vi "BORRADO_MEJORADO.vi"(9 "MB LIBRE OK":i64, 11 "MB Minimo de Memoria libre":i64) -> ()   [LabVIEW 2015]
panel:
  out "deleted path":path
  out "x > y?":bool
  out "deleted portion":path
  out "last mod":timestamp
  in  "error in":errorcluster
  out "error out 2":errorcluster
  out "Array 4":bool[](array[boolean])
  out "All Files in Dir 4":path[](array[path])
  out "double precision float 6":dbl
  out "double precision float 5":dbl
  out "x-y 3":dbl
  out "date string 3":string
  out "time string 5":string
  out "time string 7":string
  out "Array 3":timestamp[](array[timestamp])
  out "size 3":i64
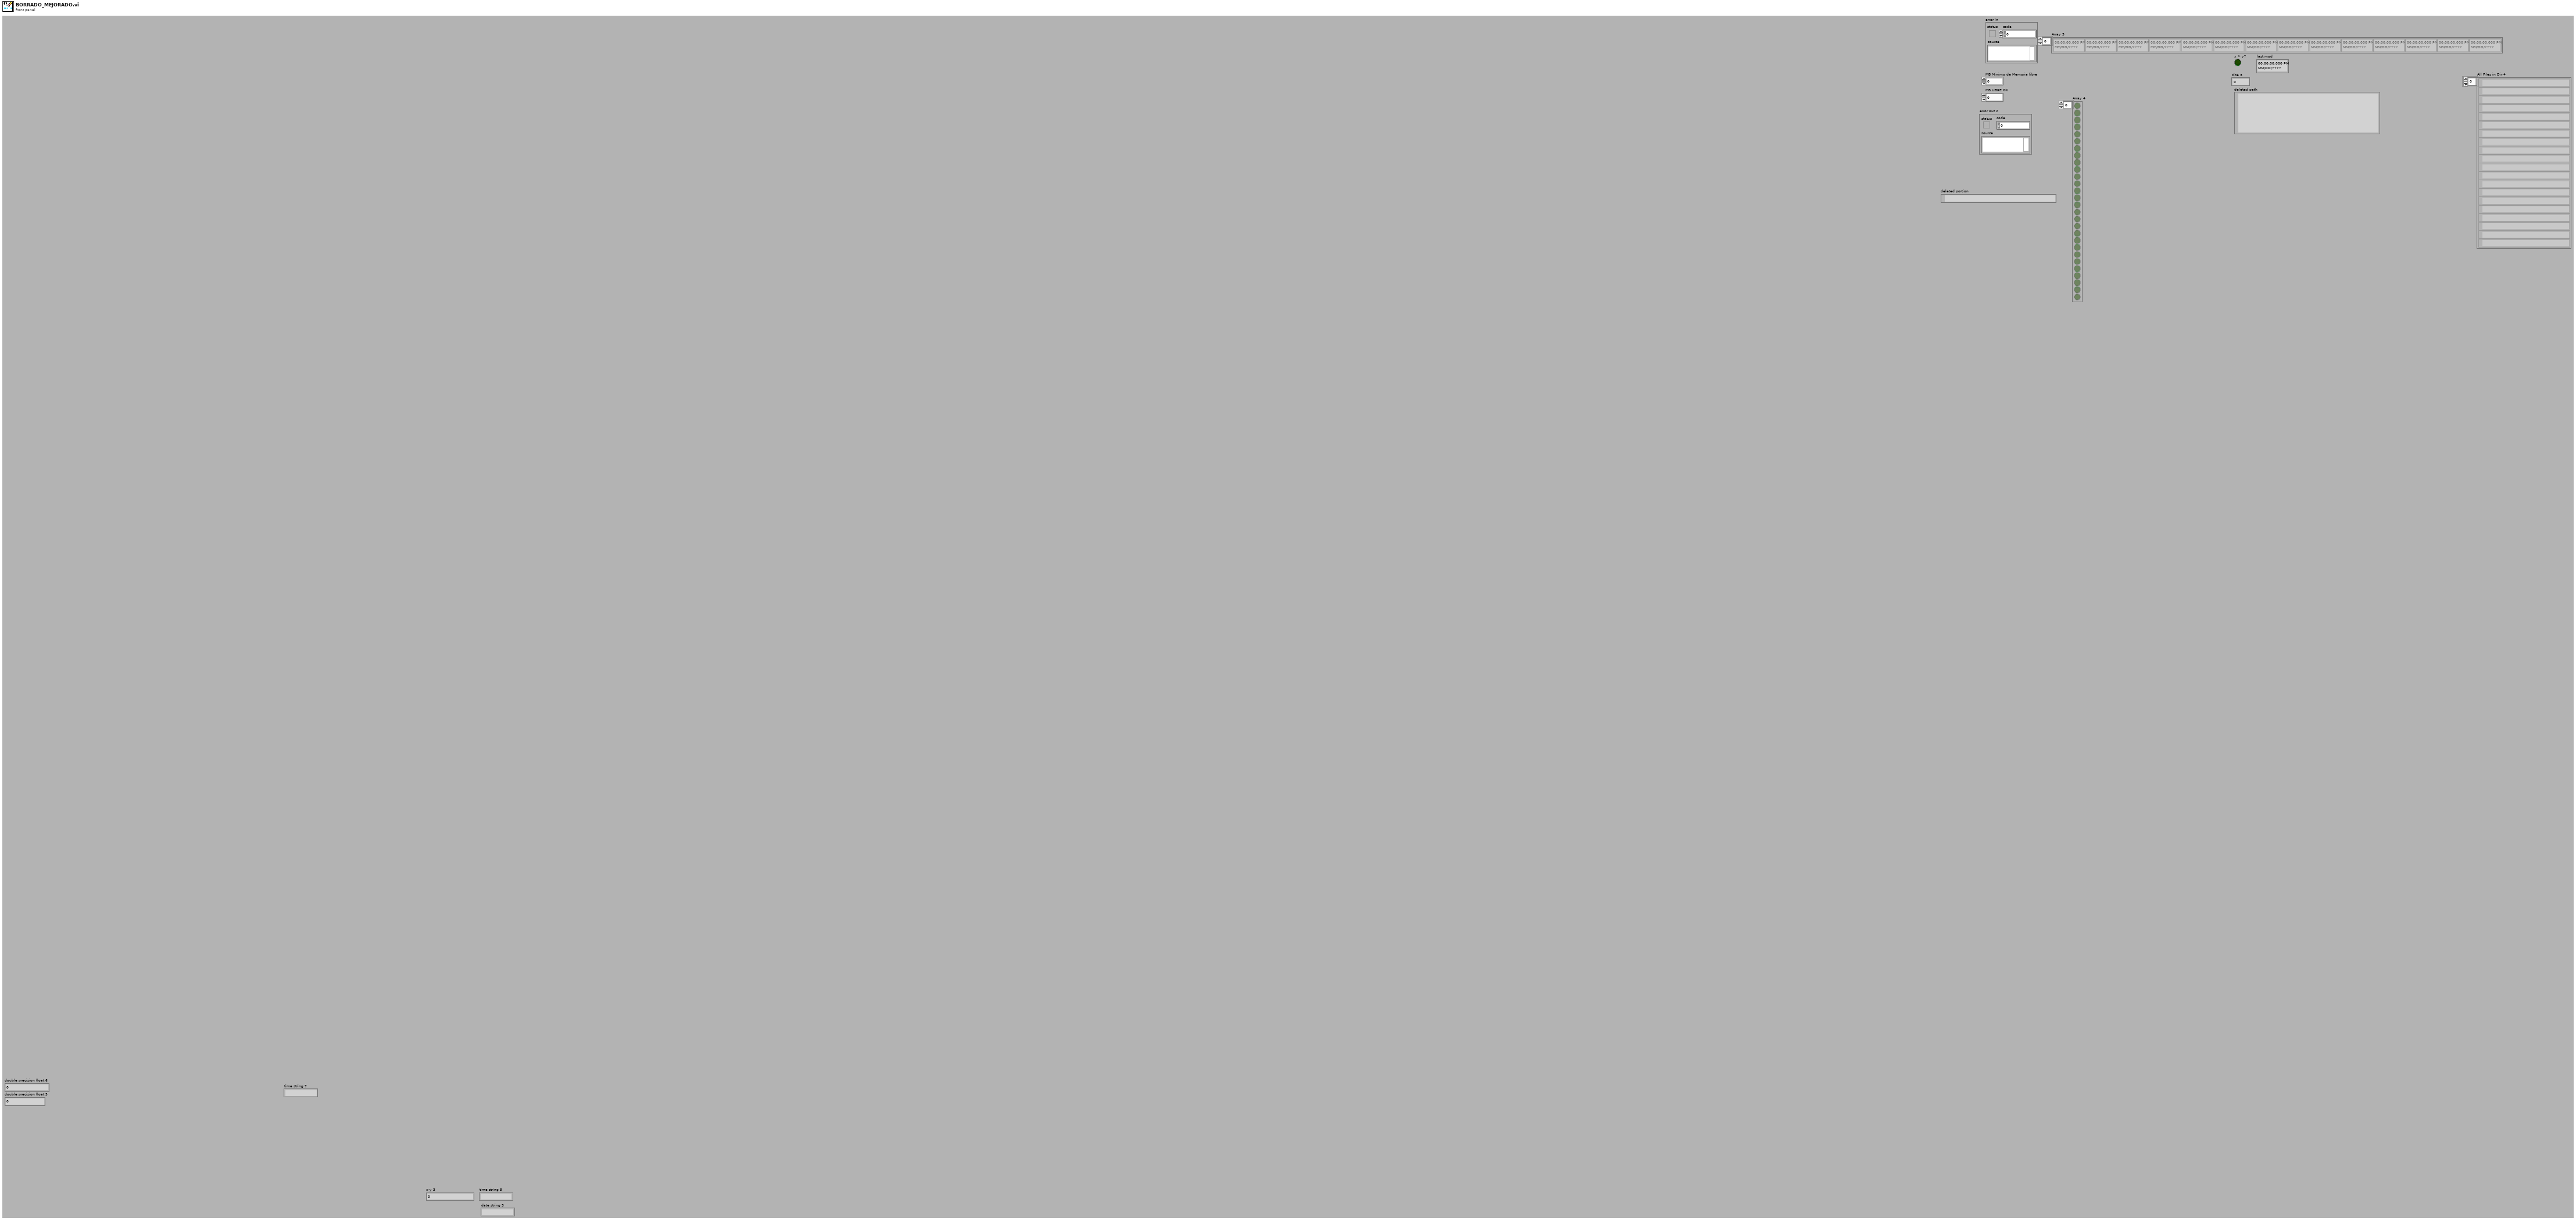
[diagram p1: front panel]
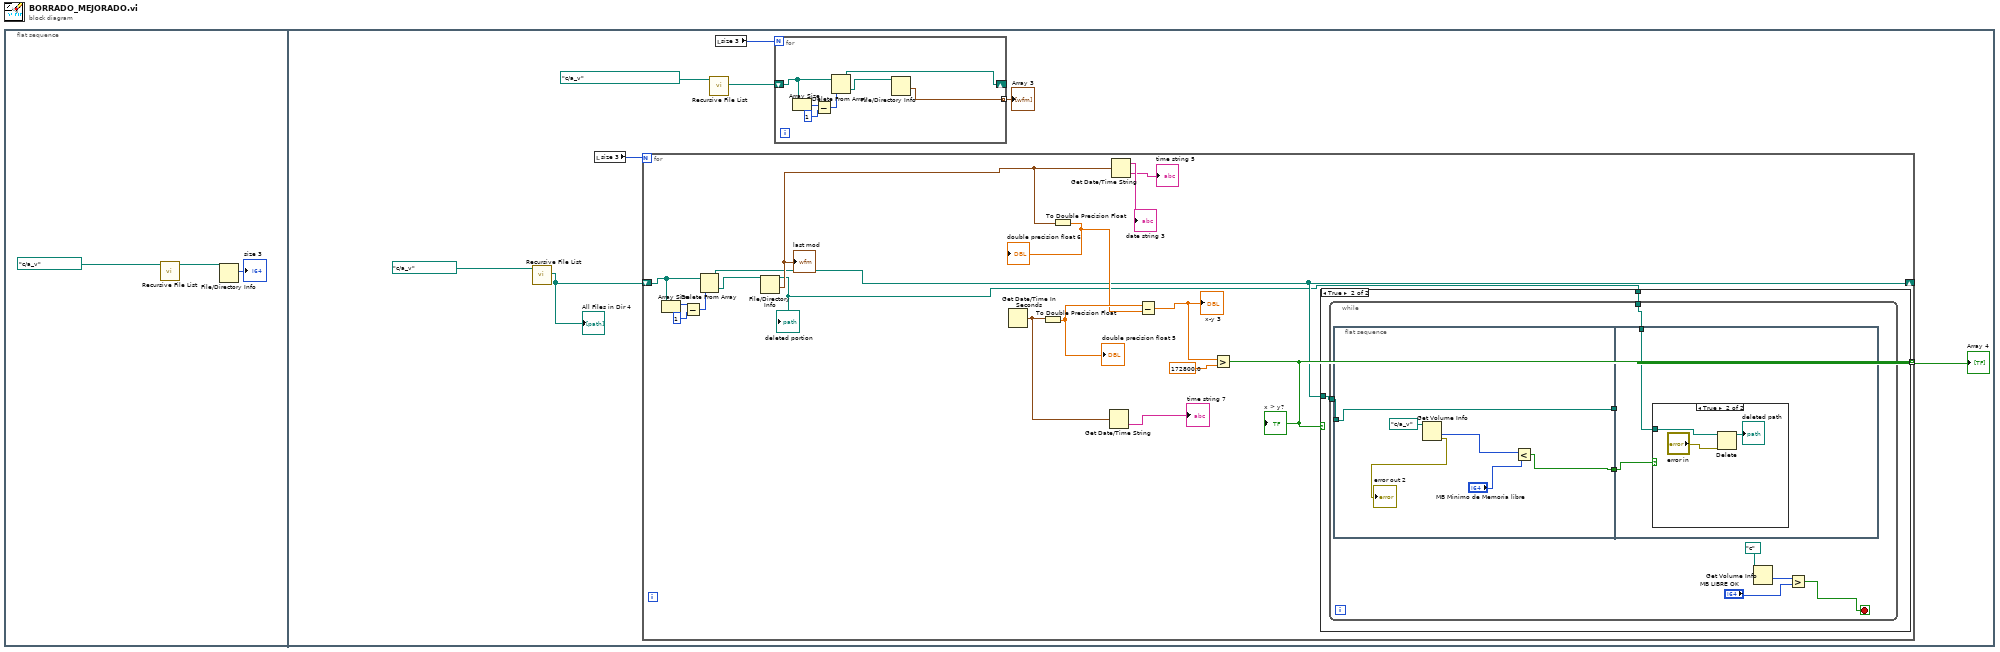
[diagram p0: block diagram]
diagram:
  n1 = flat-sequence {
    frame #0 {
      n2 = call <vilib>:"Recursive File List.vi"("Folder Path"=path "c:/a_v" ("path")) -> ("dup Folder Path"=w2:path)  [unwired: 6 in, 4 out]
      n3 = File/Directory Info(path=w2) -> (size=→"size 3":i64)  [unwired: 1 in, 6 out]
    }
    frame #1 {
      n4 = call <vilib>:"Recursive File List.vi"("Folder Path"=path "c:/a_v" ("path")) -> ("All Files in Dir"=w9:path[])  [unwired: 6 in, 4 out]
      "All Files in Dir 4" <- w9
      n5 = local read "size 3"() -> (w11:i64)
      n6 = for {
        N: w11 -> [_]
        shift-right: [w13] -> _
        shift-left: w9 -> [w24]
        tunnel: [w14] -> w10 mode=indexing
        n7 = Array Size(array=w24) -> (size(s)=w25:i32)
        n8 = Subtract(x=w25, y=1 ("length")) -> (x-y=w27:i32)
        n9 = Delete From Array(array=w24, index=w27) -> (deleted portion=w12:path, array with subset deleted=w13:path[])  [unwired: 1 in]
        "deleted portion" <- w12
        n10 = File/Directory Info(path=w12) -> (last mod=w15:timestamp)  [unwired: 1 in, 6 out]
        "last mod" <- w15
        n11 = Get Date/Time In Seconds() -> (seconds since 1Jan1904=w19:timestamp)
        n12 = To Double Precision Float(number=w19) -> (double precision float=w22:dbl)
        "double precision float 5" <- w22
        n13 = To Double Precision Float(number=w15) -> (double precision float=w21:dbl)
        "double precision float 6" <- w21
        n14 = Get Date/Time String(seconds (now)=w19) -> (time string=→"time string 7":string)  [unwired: 2 in, 1 out]
        n15 = Get Date/Time String(seconds (now)=w15) -> (date string=→"date string 3":string, time string=→"time string 5":string)  [unwired: 2 in]
        n16 = Subtract(x=w22, y=w21) -> (x-y=w17:dbl)
        "x-y 3" <- w17
        n17 = Greater?(x=w17, y=172800.0) -> (0:w14:bool)
        "x > y?" <- w14
        n18 = case shown="True" w14 {
          tunnel: w13 -> [_ w29]
          tunnel: w12 -> [_ w28]
          frame False {
          }
          frame True {
            n19 = while {
              tunnel: w29 -> [w35]
              tunnel: w28 -> [w34]
              stop <- w30 stop-if-true
              n20 = flat-sequence {
                tunnel: w35 -> [w40]
                tunnel: [w40] -> w37
                tunnel: [w39] -> w36
                tunnel: w37 -> [_]
                tunnel: w36 -> [w45]
                tunnel: w34 -> [w44]
                frame #0 {
                  n21 = Get Volume Info(11:path "c:/a_v" ("path")) -> (0:→"error out 2":errorcluster, 1:w43:i64)  [unwired: 1 in, 4 out]
                  n22 = Less?(x=w43, y="MB Minimo de Memoria libre") -> (x < y?=w39:bool)
                }
                frame #1 {
                  n23 = case shown="True" w45 {
                    tunnel: w44 -> [_ w47]
                    frame False {
                    }
                    frame True {
                      n24 = Delete(path (use dialog)=w47, error in="error in") -> (deleted path=→"deleted path":path)  [unwired: 3 in, 2 out]
                    }
                  }
                }
              }
              n25 = Get Volume Info(11:path "c:/" ("path")) -> (1:w32:i64)  [unwired: 1 in, 5 out]
              n26 = Greater?(x=w32, y="MB LIBRE OK") -> (0:w30:bool)
            }
          }
        }
      }
      "Array 4" <- w10
      n27 = call <vilib>:"Recursive File List.vi"("Folder Path"=path "c:/a_v" ("path")) -> ("All Files in Dir"=w5:path[])  [unwired: 6 in, 4 out]
      n28 = local read "size 3"() -> (w6:i64)
      n29 = for {
        N: w6 -> [_]
        shift-right: [w50] -> _
        shift-left: w5 -> [w51]
        tunnel: [w49] -> w7 mode=indexing
        n30 = Array Size(array=w51) -> (size(s)=w53:i32)
        n31 = Subtract(x=w53, y=1 ("length")) -> (x-y=w55:i32)
        n32 = Delete From Array(array=w51, index=w55) -> (deleted portion=w52:path, array with subset deleted=w50:path[])  [unwired: 1 in]
        n33 = File/Directory Info(path=w52) -> (last mod=w49:timestamp)  [unwired: 1 in, 6 out]
      }
      "Array 3" <- w7
    }
  }
